vi "Populate Fields.vi"(8 "error in (no error)":errorcluster, 10 "Field Name Array (All)":string[](array[string]), 11 "Form Model in":refnum<class "Form Model.lvclass">) -> (0 "error out":errorcluster, 3 "Form Model out":refnum<class "Form Model.lvclass">)   [LabVIEW 2020, in "Form Model.lvlib" / "Form Model.lvclass"]
uses:
  Form Model.lvclass
  Form Model.lvclass/Form Model.ctl
  Forms Controller/Panel Form Controller Messages/Populate Field Msg/Populate Field Msg.lvclass/Populate Field Msg.ctl
  <vilib>/ActorFramework/Message Enqueuer/Message Enqueuer.lvclass/Message Enqueuer.ctl
  <vilib>/ActorFramework/Message Enqueuer/Enqueue.vi
  Forms Controller/Panel Form Controller Messages/Populate Field Msg/Populate Field Msg.lvclass
  C:/Program Files (x86)/National Instruments/LabVIEW 2020/vi.lib/ActorFramework/Message/Message.lvclass
  <vilib>/ActorFramework/Message Priority Queue/Priority Enqueue.vi
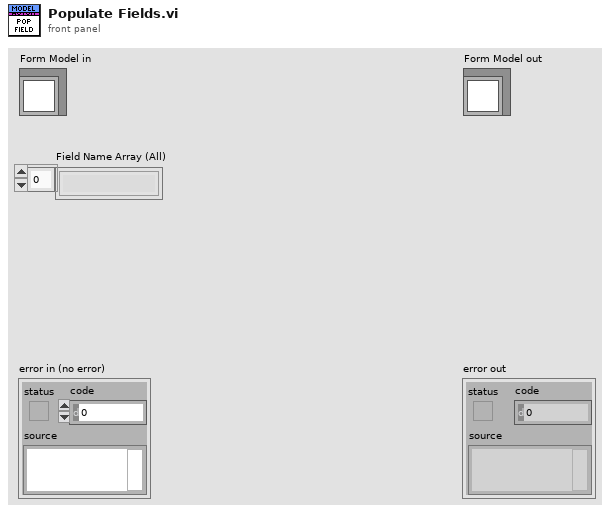
[diagram p1: front panel]
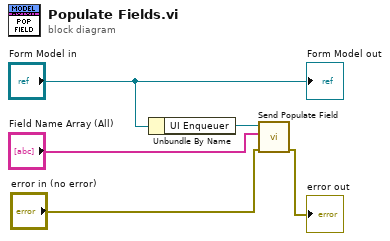
[diagram p0: block diagram]
diagram:
  n1 = Unbundle By Name("Form Model in") -> ("UI Enqueuer"=w4:refnum<class "Message Enqueuer.lvclass">)
  n2 = call "Send Populate Field.vi"("error in (no error)"="error in (no error)", "Field Name Array (All)"="Field Name Array (All)", "Message Enqueuer"=w4) -> ("error out"=→"error out":errorcluster)  [unwired: 7 in, 1 out]
  "Form Model out" <- "Form Model in"
